vi "Local gradient.vi"(6 "FFT allocated?":bool, 8 "Sizes":T1, 9 "FFT":T2, 10 "R":dbl, 11 "Image":dbl[][](array[numeric])) -> (1 "Gy":dbl[][](graph), 2 "Gx":dbl[][](graph), 3 "G":dbl[][](graph))   [LabVIEW 2015]
doc: "This vi calculates local gradients of the image\n\nINPUT:\n Im - input image\n R - radius of the window (should be >0.5)\n FFT, Sizes - Fourier transforms and sizes obtained from Local gradient preallocation\n \n OUTPUT:\n G - magnitude of local gradients\n Gx,Gy - horizontal and vertical local gradients\n \n Author: Anatolii Kashchuk"
uses:
  <vilib>/Analysis/2dsp.llb/2D Real FFT.vi
  <vilib>/Analysis/2dsp.llb/2D Inverse Real FFT.vi
  <vilib>/Analysis/NI_AALPro.lvlib
panel:
  in  "Output TAB":enum32{"Output parameters"}(tab)
  in  "Input TAB":enum32{"Input parameters"}(tab)
  out "Input image":dbl[][](graph)
  # "This vi finds local gradients of the image\nAuthor: Anatolii Kashchuk"
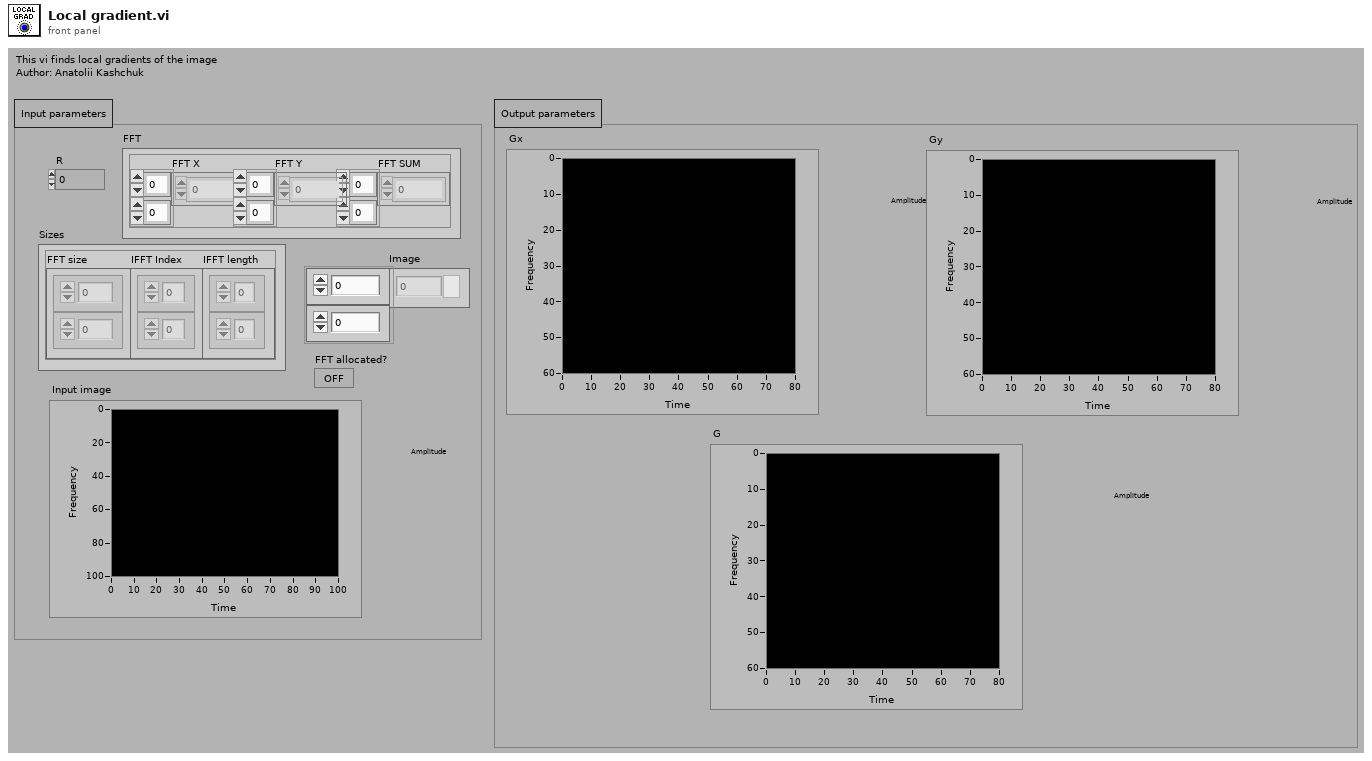
[diagram p1: front panel]
types:
  T1 = cluster{"FFT size":u32[], "IFFT Index":i32[], "IFFT length":u32[]}
  T2 = cluster{"FFT SUM":cdb[][], "FFT X":cdb[][], "FFT Y":cdb[][]}
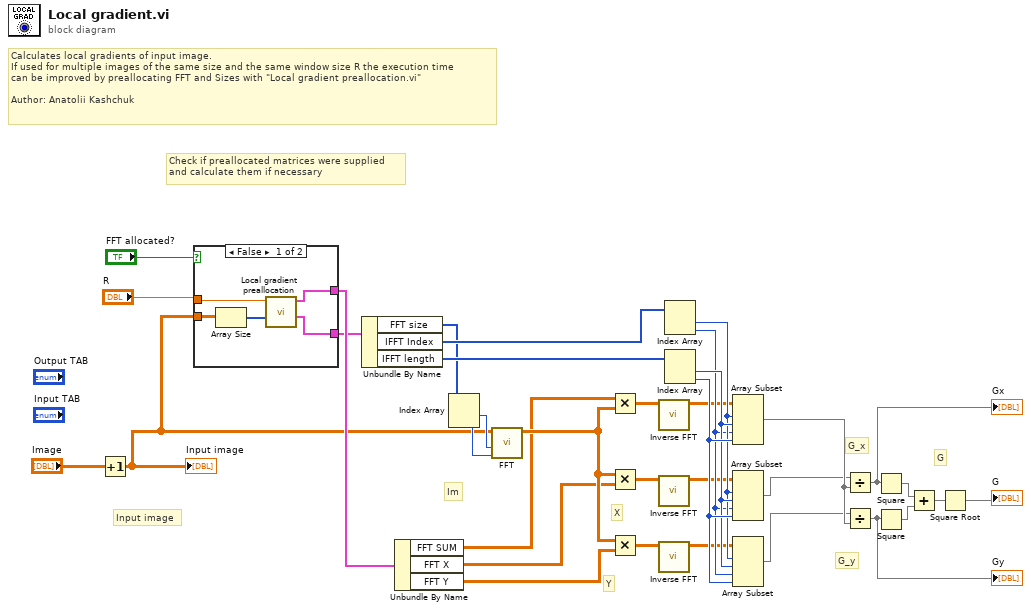
[diagram p0: block diagram]
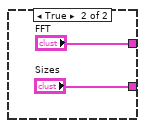
[diagram p2: hidden frame]
diagram:
  # "G"
  # "Input image"
  # "Im"
  # "X"
  # "Y"
  # "G_x"
  # "G_y"
  # "Calculates local gradients of input image. \nIf used for multiple images of the same size and the same window size R the execution time \ncan be improved by preallocating FFT and Sizes with \"Local gradient preallocation.vi\"\n\nAuthor: Anatolii Kashchuk"
  # "Check if preallocated matrices were supplied\nand calculate them if necessary"
  n1 = Increment(x="Image") -> (x+1=w1:dbl[][])
  "Input image" <- w1
  n2 = case shown="False" "FFT allocated?" {
    tunnel: "R" -> [w39 _]
    tunnel: [w38 "FFT"] -> w17
    tunnel: [w37 "Sizes"] -> w16
    tunnel: w1 -> [w36 _]
    frame False {
      n3 = Array Size(array=w36) -> (size(s)=w35:i32[])
      n4 = call "Local gradient preallocation.vi"("Image size"=w35, "R"=w39) -> ("Sizes"=w37:T1, "FFT"=w38:T2)  [unwired: 8 in]
    }
    frame True {
    }
  }
  n5 = Unbundle By Name(w16) -> ("FFT size"=w13:u32[], "IFFT Index"=w15:i32[], "IFFT length"=w14:u32[])
  n6 = Unbundle By Name(w17) -> ("FFT SUM"=w10:cdb[][], "FFT X"=w9:cdb[][], "FFT Y"=w8:cdb[][])
  n7 = Index Array(array=w13) -> (element #1=w12:u32, element #2=w11:u32)  [unwired: 2 in]
  n8 = call-poly <vilib>:"FFT.vi"("n"=w11, "m"=w12, "X"=w1) -> ("FFT {X}"=w22:cdb[][])  [unwired: 7 in, 1 out]
  n9 = Multiply(x=w10, y=w22) -> (x*y=w21:cdb[][])
  n10 = Multiply(x=w22, y=w9) -> (x*y=w23:cdb[][])
  n11 = Multiply(x=w22, y=w8) -> (x*y=w24:cdb[][])
  n12 = call-poly <vilib>:"Inverse FFT.vi"("FFT {X}"=w21) -> ("X"=w20:dbl[][])  [unwired: 9 in, 1 out]
  n13 = call-poly <vilib>:"Inverse FFT.vi"("FFT {X}"=w23) -> ("X"=w19:dbl[][])  [unwired: 9 in, 1 out]
  n14 = call-poly <vilib>:"Inverse FFT.vi"("FFT {X}"=w24) -> ("X"=w18:dbl[][])  [unwired: 9 in, 1 out]
  n15 = Index Array(array=w15) -> (element #1=w27:i32, element #2=w26:i32)  [unwired: 2 in]
  n16 = Index Array(array=w14) -> (element #1=w28:u32, element #2=w29:u32)  [unwired: 2 in]
  n17 = Array Subset(array=w20, index (row)=w27, length (row)=w28, index (col)=w26, length (col)=w29) -> (w25:dbl[][])
  n18 = Array Subset(array=w19, index (row)=w27, length (row)=w28, index (col)=w26, length (col)=w29) -> (w3:dbl[][])
  n19 = Array Subset(array=w18, index (row)=w27, length (row)=w28, index (col)=w26, length (col)=w29) -> (w4:dbl[][])
  n20 = Divide(x=w3, y=w25) -> (x/y=w7:dbl[][])
  "Gx" <- w7
  n21 = Divide(x=w4, y=w25) -> (x/y=w6:dbl[][])
  "Gy" <- w6
  n22 = Square(x=w7) -> (x^2=w33:dbl[][])
  n23 = Square(x=w6) -> (x^2=w31:dbl[][])
  n24 = Add(x=w33, y=w31) -> (x+y=w32:dbl[][])
  n25 = Square Root(x=w32) -> (sqrt(x)=→"G":dbl[][])
